vi "Main.vi"() -> ()   [LabVIEW 2018]
doc: "This project is based on the Queued Message Handler template.\n\nThe Event Handling Loop generates messages based on user interface actions.\n\nThe Message Handling Loop processes messages generated by the Event Handling Loop, or by other messages. There are also Acquisition and Logging message handling loop subVIs, and a chart updating loop."
uses:
  Settings/Settings.ctl
  Acquisition/Hardware Configuration.ctl
  Logging/Logging Configuration.ctl
  controls/UI RefNums.ctl
  Analysis/Global Tube Length.vi
  support/Global Offsets.vi
  Settings/Settings.lvlib
  support/User Event - Stop/User Event - Stop.lvlib
  support/Message Queue/Message Queue.lvlib
  <vilib>/Analysis/NI_AALBase.lvlib
  Logging/Logging.lvlib
  Analysis/Analysis.lvlib
  Acquisition/Acquisition.lvlib
panel:
  out "Long Offset":string
  out "Mid Offset":string
  out "Short Offset":string
  out "Timer":dbl(knob) scale=0.0..300.0
  in  "Long":dbl format="%_5g"
  in  "Mid":dbl format="%_5g"
  in  "Short":dbl format="%.4g"
  out "System Log":string
  out "L":bool
  out "M":bool
  in  "Collar":dbl format="%.4g"
  out "Thermistors":cluster{i32[], "Temp Out":dbl[]}(graph)
  in  "Exit":bool
  in  "Settings":bool
  out "RS232 Buffer":string
  out "S":bool
  in  "Start":bool
  out "Average Temperature Time Series":dbl(graph)
  out "Ring Time":waveform(dbl)(graph)
  # "Offsets"
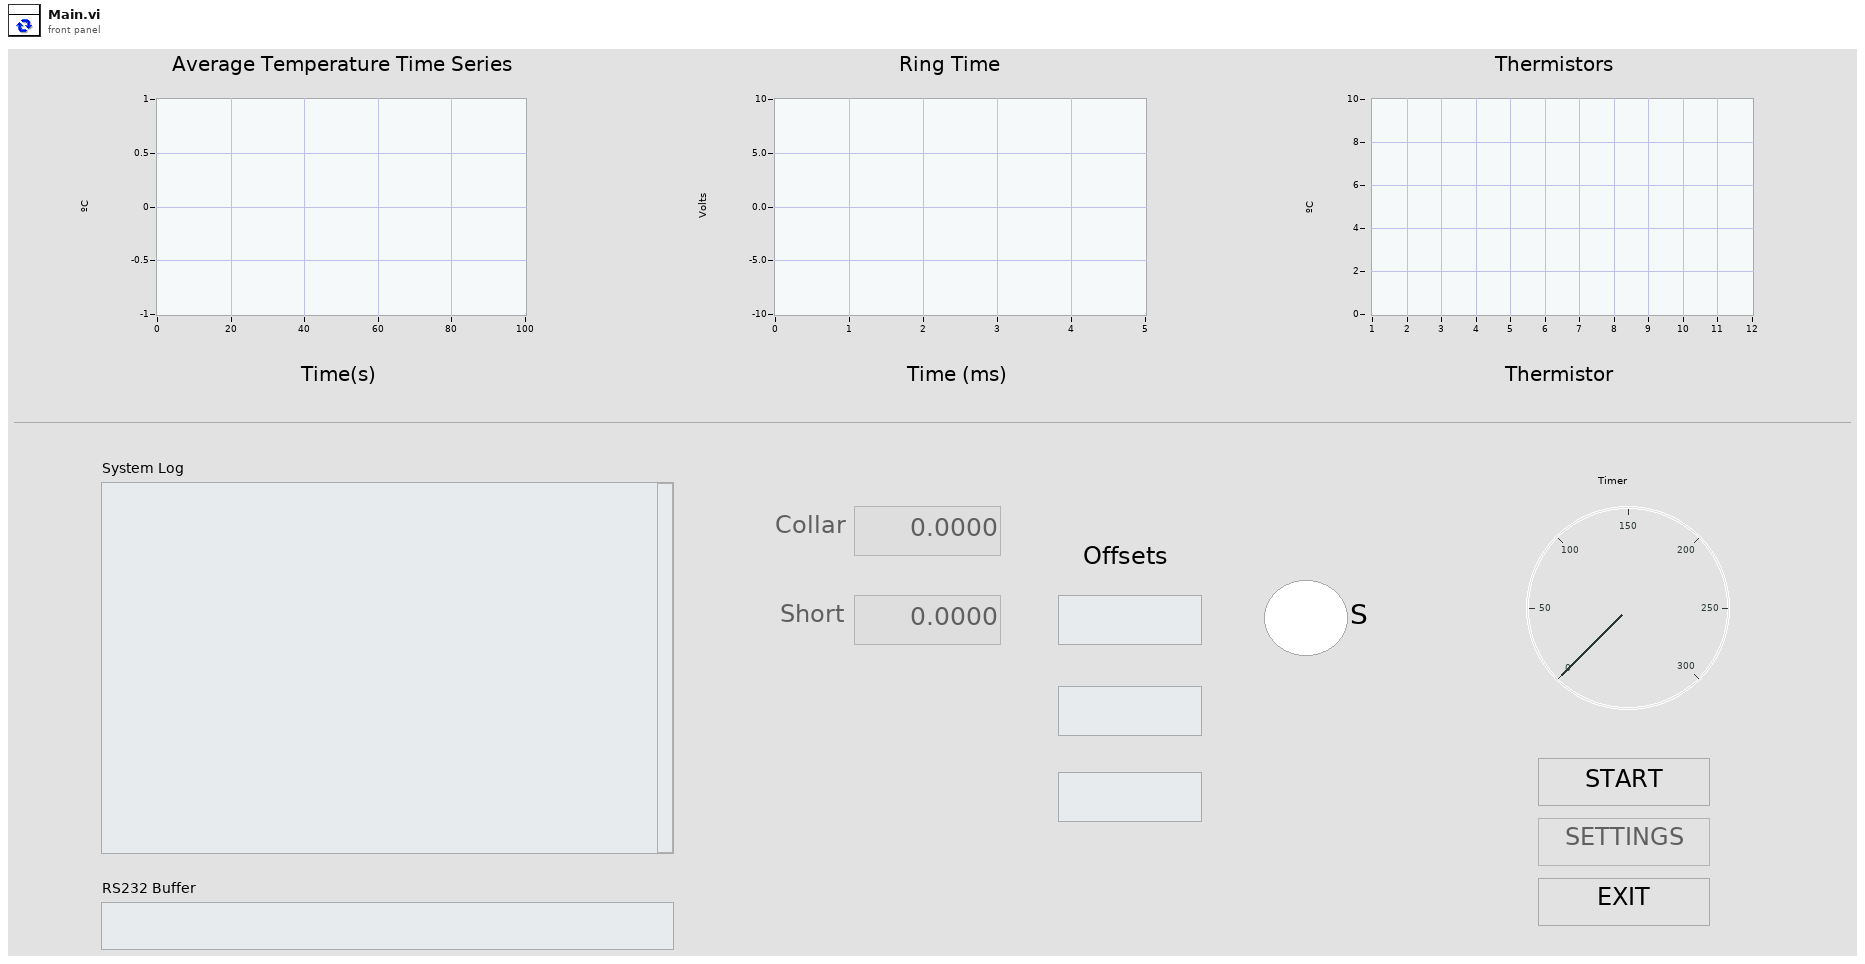
[diagram p1: front panel]
types:
  T1 = typedef "Settings.ctl" = cluster{"Hardware Configuration":T2, "Logging Configuration":T3, "UI RefNums":T4, "Meta Data":cluster{"Calibration Location":string, "Operator Name":string, "Sensor SN":string, "Cal Tube SN":string, "Comments":string, "Start Time":string}}
  T2 = typedef "Acquisition.lvlib/Hardware Configuration.ctl" = cluster{"DAQmx AI Channels":tag, "Aquatrak COM Port":refnum<visa-resource-name>, "Ring Time Task":refnum<k21>}
  T3 = typedef "Logging.lvlib/Logging Configuration.ctl" = cluster{"Log File Base Path":path, "Data Log Refnum":refnum<k1>}
  T4 = typedef "UI RefNums.ctl" = cluster{"Start Ref":refnum<vi>, "Settings Ref":refnum<vi>, "Exit Ref":refnum<vi>, "System Log Ref":refnum<vi>, "RS232 Buffer Ref":refnum<vi>, "Ringtime Ref":refnum<vi>, "Avg Temp Ref":refnum<vi>, "Thermistors Ref":refnum<vi>, "Collar Meas Ref":refnum<vi>, "Short Meas Ref":refnum<vi>, "Mid Meas Ref":refnum<vi>, "Long Meas Ref":refnum<vi>, "Short LED Ref":refnum<vi>, "Mid LED Ref":refnum<vi>, "Long LED Ref":refnum<vi>, "Short Offset Ref":refnum<vi>, "Mid Offset Ref":refnum<vi>, "Long Offset Ref":refnum<vi>, "Timer Ref":refnum<vi>}
  T5 = typedef "Message Queue.lvlib/All Message Queues.ctl" = cluster{"UI":refnum<queue>, "Acquisition":refnum<queue>, "Logging":refnum<queue>, "Analyze":refnum<queue>, "Data Notifier":refnum<notifier>, "Data Queue":refnum<queue>}
  T6 = typedef "Acquired Data.ctl" = cluster{"Average Range":dbl, "Temp Array":dbl[][], "Cal Counts":i32, "Range Counts":i32, "Timestamp (UTC)":string}
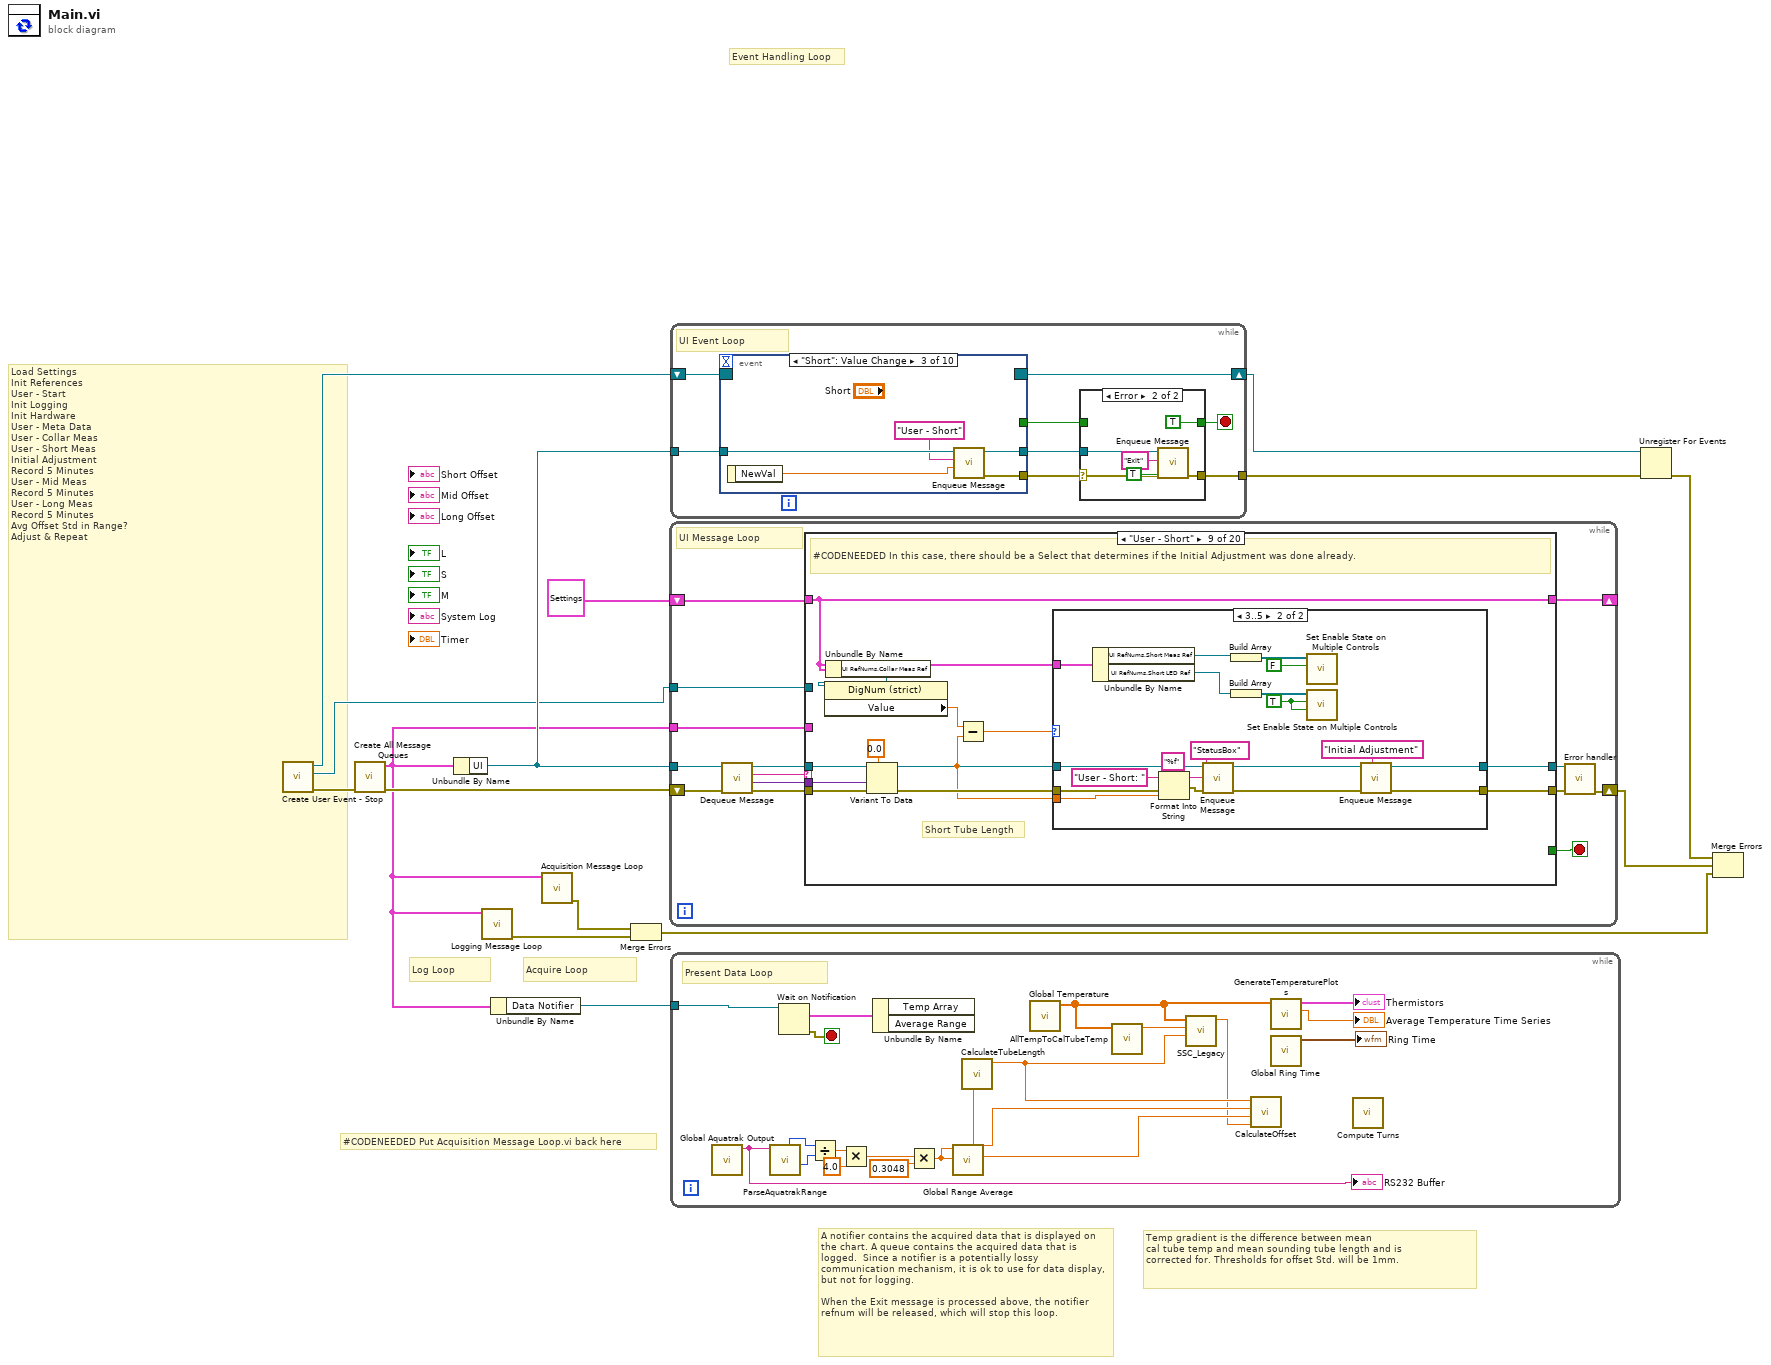
[diagram p0: block diagram]
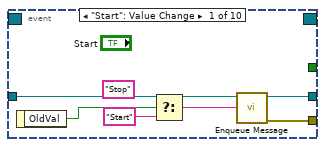
[diagram p3: hidden frame]
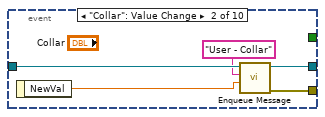
[diagram p4: hidden frame]
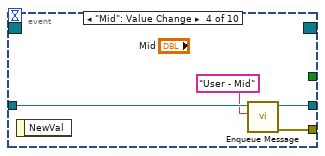
[diagram p5: hidden frame]
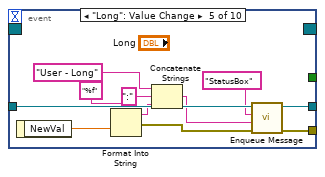
[diagram p6: hidden frame]
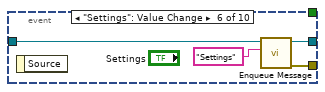
[diagram p7: hidden frame]
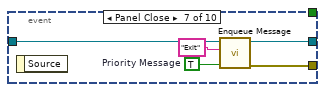
[diagram p8: hidden frame]
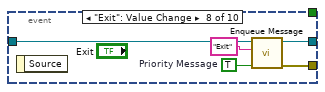
[diagram p9: hidden frame]
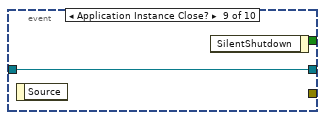
[diagram p10: hidden frame]
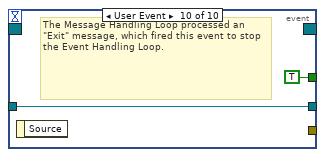
[diagram p11: hidden frame]
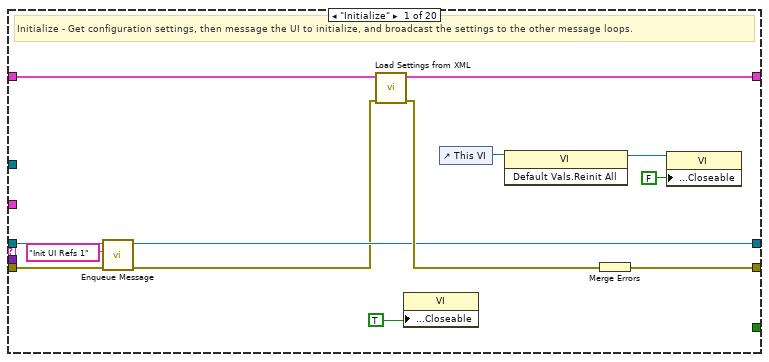
[diagram p12: hidden frame]
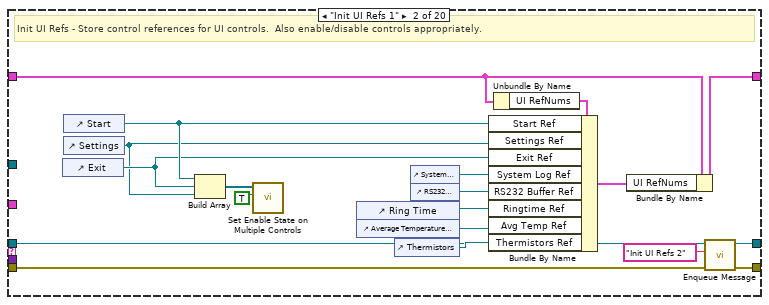
[diagram p13: hidden frame]
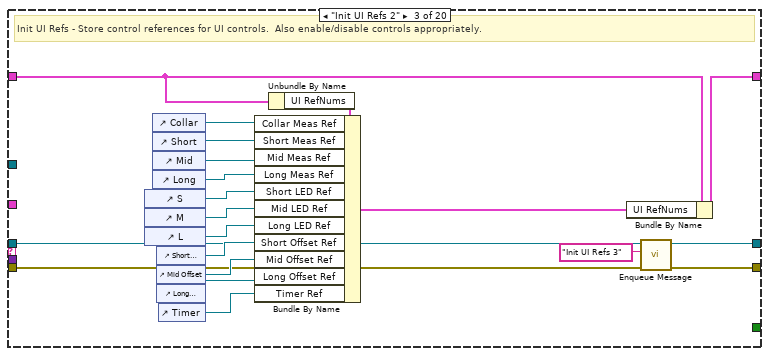
[diagram p14: hidden frame]
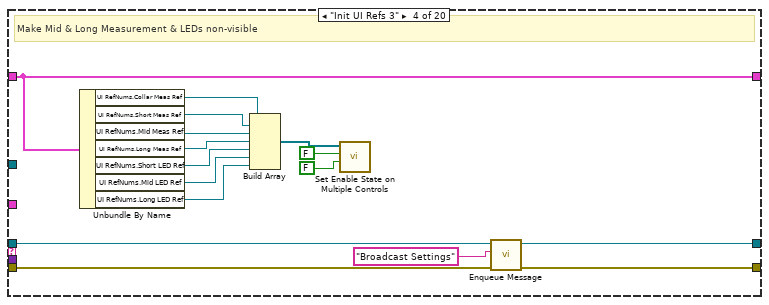
[diagram p15: hidden frame]
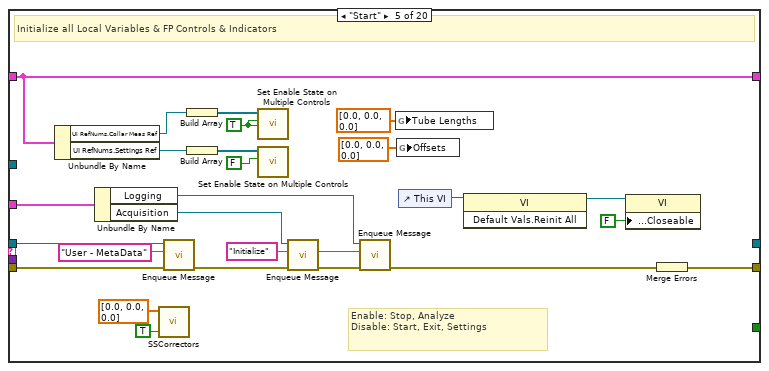
[diagram p16: hidden frame]
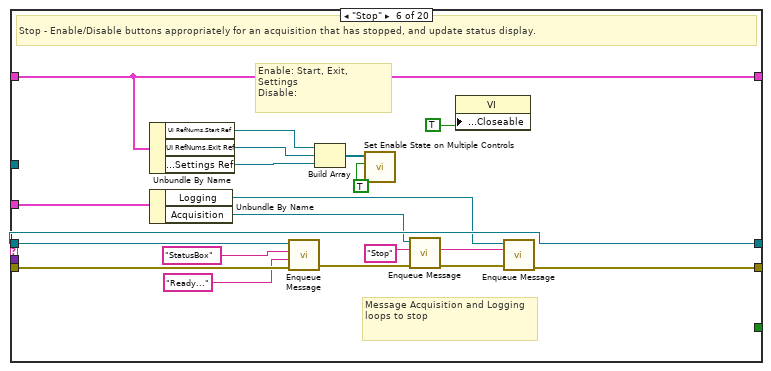
[diagram p17: hidden frame]
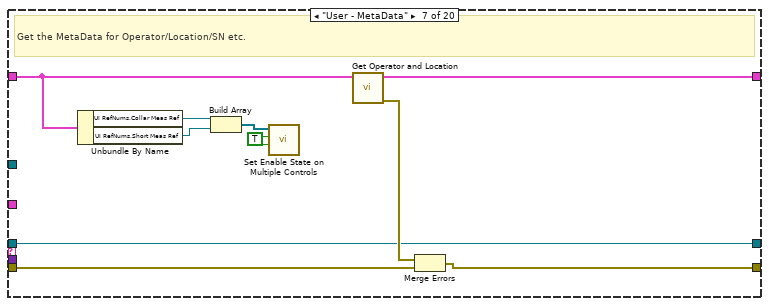
[diagram p18: hidden frame]
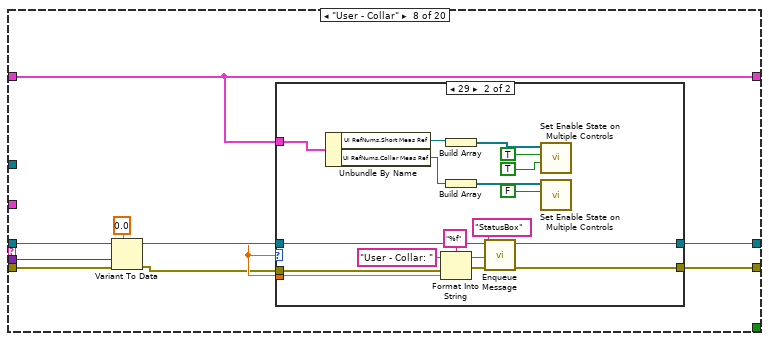
[diagram p19: hidden frame]
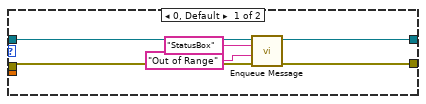
[diagram p20: hidden frame]
diagram:
  # "#CODENEEDED Put Acquisition Message Loop.vi back here"
  # "Acquire Loop"
  # "Log Loop"
  # "Event Handling Loop"
  # "Temp gradient is the difference between mean\ncal tube temp and mean sounding tube length and is \ncorrected for. Thresholds for offset Std. will be 1mm."
  # "A notifier contains the acquired data that is displayed on the chart. A queue contains the acquired data that is logged.  Since a notifier is a potentially lossy communication mechanism, it is ok to use for data display, but not for logging.\n\nWhen the Exit message is processed above, the notifier refnum will be released, which will stop this loop."
  # "Load Settings\nInit References\nUser - Start\nInit Logging\nInit Hardware\nUser - Meta Data\nUser - Collar Meas\nUser - Short Meas\nInitial Adjustment\nRecord 5 Minutes\nUser - Mid Meas\nRecord 5 Minutes\nUser - Long Meas\nRecord 5 Minutes\nAvg Offset Std in Range?\nAdjust & Repeat"
  n1 = call "Create User Event - Stop.vi"() -> ("error out"=w11:errorcluster, "User Event - Stop"=w5:refnum<user-event>, "Stop Event Registration Refnum"=w12:refnum<event-registration>)  [unwired: 9 in]
  n2 = call "Create All Message Queues.vi"("error in (no error)"=w11) -> ("error out"=w8:errorcluster, "Message Queues out"=w2:T5)  [unwired: 9 in]
  n3 = Unbundle By Name(w2) -> ("UI"=w15:refnum<queue>)
  n4 = call "Logging Message Loop.vi"("Message Queues"=w2) -> ("error out"=w4:errorcluster)  [unwired: 10 in]
  n5 = Unbundle By Name(w2) -> ("Data Notifier"=w6:refnum<notifier>)
  n6 = call "Acquisition Message Loop.vi"("Message Queues"=w2) -> ("error out"=w1:errorcluster)  [unwired: 10 in]
  n7 = Merge Errors(w1, w4) -> (w3:errorcluster)
  n8 = while {
    tunnel: w15 -> [w22]
    tunnel: w5 -> [w28]
    shift-right: [w19] -> w14
    shift-left: w8 -> [w27]
    shift-right: [w17] -> _
    shift-left: T1 {"Hardware Configuration"={"DAQmx AI Channels"="", "Aquatrak COM Port"="", "Ring Time Task"=""}, "Logging Configuration"={"Log File Base Path"=path "", "Data Log Refnum"=refnum}, "UI RefNums"={"Start Ref"=refnum, "Settings Ref"=refnum, "Exit Ref"=refnum, "System Log Ref"=refnum, "RS232 Buffer Ref"=refnum, "Ringtime Ref"=refnum, "Avg Temp Ref"=refnum, "Thermistors Ref"=refnum, "Collar Meas Ref"=refnum, "Short Meas Ref"=refnum, "Mid Meas Ref"=refnum, "Long Meas Ref"=refnum, "Short LED Ref"=refnum, "Mid LED Ref"=refnum, "Long LED Ref"=refnum, "Short Offset Ref"=refnum, "Mid Offset Ref"=refnum, "Long Offset Ref"=refnum, "Timer Ref"=refnum}, "Meta Data"={"Calibration Location"="", "Operator Name"="", "Sensor SN"="", "Cal Tube SN"="", "Comments"="", "Start Time"=""}} ("Settings") -> [w21]
    tunnel: w2 -> [w16]
    stop <- w29 stop-if-true
    # "UI Message Loop"
    n9 = call "Dequeue Message.vi"("error in (no error)"=w27, "Message Queue"=w22) -> ("error out"=w26:errorcluster, "Message Data"=w24:variant, "Message"=w25:string, "dup Message Queue"=w23:refnum<queue>)  [unwired: 6 in]
    n10 = case "Message Cases" shown="\"User - Short\"" w25 {
      selector: w25 -> [_ _ _ _ _ _ _ _ _ _ _ _ _ _ _ _ _ _ _ w367]
      tunnel: w23 -> [w39 w46 w65 w91 w109 w140 w146 w159 w195 w228 w238 w265 w304 w306 w313 w327 w338 w354 w358 w362]
      tunnel: w26 -> [w38 w45 w64 w90 w108 w139 w149 w156 w192 w223 w235 w268 w305 w308 w316 w331 w339 w350 w361 _]
      tunnel: [w37 w43 w62 w88 w120 w131 w147 w157 w193 w222 w236 w268 w305 w308 w315 w332 w336 w347 w360 w365] -> w18
      tunnel: [_ _ _ _ _ _ _ _ _ _ _ _ _ _ _ _ _ TRUE _ _] -> w29
      tunnel: w24 -> [_ _ _ _ _ _ _ w154 w190 _ w233 _ _ _ _ w330 _ _ _ _]
      tunnel: w28 -> [_ _ _ _ _ _ _ _ _ _ _ _ _ _ _ _ _ w356 _ _]
      tunnel: w21 -> [w42 w55 w80 w97 w113 w127 w144 w151 w186 w226 w231 w270 w303 w307 w312 w326 w340 w355 w359 w363]
      tunnel: [w34 w44 w63 w89 _ w140 w146 w158 w194 w228 w237 w265 w304 w306 w313 w327 w333 _ w358 w362] -> w20
      tunnel: [w40 w54 w79 w97 w113 w127 w148 w151 w186 w226 w231 w270 w303 w307 w312 w326 w335 w355 w359 w363] -> w17
      tunnel: w16 -> [_ _ _ _ w106 w125 _ _ _ w225 _ _ _ _ w311 _ _ w345 _ _]
      frame "Initialize" {
        # "Initialize - Get configuration settings, then message the UI to initialize, and broadcast the settings to the other message loops."
        n11 = call "Enqueue Message.vi"("error in (no error)"=w38, "Message"="Init UI Refs 1", "Message Queue"=w39) -> ("error out"=w33:errorcluster, "dup Message Queue"=w34:refnum<queue>)  [unwired: 7 in]
        n12 = call "Load Settings from XML.vi"("error in (no error)"=w33, "Settings in"=w42) -> ("error out"=w41:errorcluster, "Settings out"=w40:T1)  [unwired: 8 in]
        n13 = property class="VI"("Front Panel.Closeable"=TRUE ("Front Panel Window:Closeable")) -> ()  [unwired: 2 in, 2 out]
        n14 = control-ref of="This VI"() -> (w31:refnum<vi>)
        n15 = invoke class="VI" method="Default Vals.Reinit All"(reference=w31) -> (reference out=w30:refnum<vi>)  [unwired: 2 in, 2 out]
        n16 = Merge Errors(w41) -> (w37:errorcluster)
        n17 = property class="VI"(reference=w30, "Front Panel.Closeable"=FALSE ("Front Panel Window:Closeable")) -> ()  [unwired: 1 in, 2 out]
      }
      frame "Init UI Refs 1" {
        # "Init UI Refs - Store control references for UI controls.  Also enable/disable controls appropriately."
        n18 = control-ref of="Exit"() -> (w58:refnum<vi>)
        n19 = control-ref of="Start"() -> (w59:refnum<vi>)
        n20 = control-ref of="Settings"() -> (w57:refnum<vi>)
        n21 = Build Array(w59, w58, w57) -> (w60:refnum<vi>[])
        n22 = call "Set Enable State on Multiple Controls.vi"("Enable?"=TRUE, "Controls"=w60) -> ()  [unwired: 10 in]
        n23 = control-ref of="Ring Time"() -> (w50:refnum<vi>)
        n24 = control-ref of="Average Temperature Time Series"() -> (w49:refnum<vi>)
        n25 = control-ref of="Thermistors"() -> (w48:refnum<vi>)
        n26 = control-ref of="System Log"() -> (w52:refnum<vi>)
        n27 = control-ref of="RS232 Buffer"() -> (w51:refnum<vi>)
        n28 = Unbundle By Name(w55) -> ("UI RefNums"=w56:T4)
        n29 = Bundle By Name(cluster=w56, "Start Ref"=w59, "Settings Ref"=w57, "Exit Ref"=w58, "System Log Ref"=w52, "RS232 Buffer Ref"=w51, "Ringtime Ref"=w50, "Avg Temp Ref"=w49, "Thermistors Ref"=w48) -> (w53:T4)
        n30 = Bundle By Name(cluster=w55, "UI RefNums"=w53) -> (w54:T1)
        n31 = call "Enqueue Message.vi"("error in (no error)"=w45, "Message"="Init UI Refs 2", "Message Queue"=w46) -> ("error out"=w43:errorcluster, "dup Message Queue"=w44:refnum<queue>)  [unwired: 7 in]
      }
      frame "Init UI Refs 2" {
        # "Init UI Refs - Store control references for UI controls.  Also enable/disable controls appropriately."
        n32 = control-ref of="S"() -> (w77:refnum<vi>)
        n33 = control-ref of="M"() -> (w76:refnum<vi>)
        n34 = control-ref of="L"() -> (w75:refnum<vi>)
        n35 = control-ref of="Collar"() -> (w73:refnum<vi>)
        n36 = control-ref of="Short"() -> (w72:refnum<vi>)
        n37 = control-ref of="Mid"() -> (w71:refnum<vi>)
        n38 = control-ref of="Long"() -> (w70:refnum<vi>)
        n39 = control-ref of="Short Offset"() -> (w69:refnum<vi>)
        n40 = control-ref of="Mid Offset"() -> (w68:refnum<vi>)
        n41 = control-ref of="Long Offset"() -> (w67:refnum<vi>)
        n42 = control-ref of="Timer"() -> (w74:refnum<vi>)
        n43 = Unbundle By Name(w80) -> ("UI RefNums"=w81:T4)
        n44 = Bundle By Name(cluster=w81, "Collar Meas Ref"=w73, "Short Meas Ref"=w72, "Mid Meas Ref"=w71, "Long Meas Ref"=w70, "Short LED Ref"=w77, "Mid LED Ref"=w76, "Long LED Ref"=w75, "Short Offset Ref"=w69, "Mid Offset Ref"=w68, "Long Offset Ref"=w67, "Timer Ref"=w74) -> (w78:T4)
        n45 = Bundle By Name(cluster=w80, "UI RefNums"=w78) -> (w79:T1)
        n46 = call "Enqueue Message.vi"("error in (no error)"=w64, "Message"="Init UI Refs 3", "Message Queue"=w65) -> ("error out"=w62:errorcluster, "dup Message Queue"=w63:refnum<queue>)  [unwired: 7 in]
      }
      frame "Init UI Refs 3" {
        # "Make Mid & Long Measurement & LEDs non-visible"
        n47 = Unbundle By Name(w97) -> ("UI RefNums.Collar Meas Ref"=w82:refnum<vi>, "UI RefNums.Short Meas Ref"=w87:refnum<vi>, "UI RefNums.Mid Meas Ref"=w96:refnum<vi>, "UI RefNums.Long Meas Ref"=w95:refnum<vi>, "UI RefNums.Short LED Ref"=w94:refnum<vi>, "UI RefNums.Mid LED Ref"=w93:refnum<vi>, "UI RefNums.Long LED Ref"=w86:refnum<vi>)
        n48 = Build Array(w82, w87, w96, w95, w94, w93, w86) -> (w84:refnum<vi>[])
        n49 = call "Set Enable State on Multiple Controls.vi"("Visible?"=FALSE ("Enable?"), "Enable?"=FALSE, "Controls"=w84) -> ()  [unwired: 9 in]
        n50 = call "Enqueue Message.vi"("error in (no error)"=w90, "Message"="Broadcast Settings", "Message Queue"=w91) -> ("error out"=w88:errorcluster, "dup Message Queue"=w89:refnum<queue>)  [unwired: 7 in]
      }
      frame "Start" {
        w101 = TRUE ("Enable?")
        w117 = "Initialize" ("Message")
        # "Enable: Stop, Analyze\nDisable: Start, Exit, Settings"
        # "Initialize all Local Variables & FP Controls & Indicators"
        n51 = Unbundle By Name(w113) -> ("UI RefNums.Collar Meas Ref"=w102:refnum<vi>, "UI RefNums.Settings Ref"=w112:refnum<vi>)
        n52 = Unbundle By Name(w106) -> ("Logging"=w105:refnum<queue>, "Acquisition"=w104:refnum<queue>)
        n53 = call "SSCorrectors.vi"("Write?"=TRUE, "SSC In (meters)"=dbl[] [0.0, 0.0, 0.0]) -> ()  [unwired: 8 in, 2 out]
        n54 = call "Enqueue Message.vi"("error in (no error)"=w108, "Message"="User - MetaData", "Message Queue"=w109) -> ("error out"=w107:errorcluster)  [unwired: 7 in, 1 out]
        n55 = Build Array(w102) -> (w103:refnum<vi>[])
        n56 = Build Array(w112) -> (w111:refnum<vi>[])
        n57 = call "Set Enable State on Multiple Controls.vi"("Visible?"=w101, "Enable?"=w101, "Controls"=w103) -> ()  [unwired: 9 in]
        n58 = call "Set Enable State on Multiple Controls.vi"("Enable?"=FALSE, "Controls"=w111) -> ()  [unwired: 10 in]
        n59 = call "Enqueue Message.vi"("error in (no error)"=w107, "Message"=w117, "Message Queue"=w104) -> ("error out"=w118:errorcluster)  [unwired: 7 in, 1 out]
        n60 = call "Enqueue Message.vi"("error in (no error)"=w118, "Message"=w117, "Message Queue"=w105) -> ("error out"=w121:errorcluster)  [unwired: 7 in, 1 out]
        n61 = global write "Global Tube Length.vi" "Tube Lengths"(dbl[] [0.0, 0.0, 0.0] ("Tube Lengths")) -> ()
        n62 = global write "Global Offsets.vi" "Offsets"(dbl[] [0.0, 0.0, 0.0] ("Offsets")) -> ()
        n63 = control-ref of="This VI"() -> (w99:refnum<vi>)
        n64 = invoke class="VI" method="Default Vals.Reinit All"(reference=w99) -> (reference out=w98:refnum<vi>)  [unwired: 2 in, 2 out]
        n65 = property class="VI"(reference=w98, "Front Panel.Closeable"=FALSE ("Front Panel Window:Closeable")) -> ()  [unwired: 1 in, 2 out]
        n66 = Merge Errors(w121) -> (w120:errorcluster)
      }
      frame "Stop" {
        w128 = "Stop" ("Message")
        # "Message Acquisition and Logging loops to stop"
        # "Stop - Enable/Disable buttons appropriately for an acquisition that has stopped, and update status display."
        # "Enable: Start, Exit, Settings\nDisable:"
        n67 = Unbundle By Name(w127) -> ("UI RefNums.Start Ref"=w135:refnum<vi>, "UI RefNums.Exit Ref"=w134:refnum<vi>, "UI RefNums.Settings Ref"=w133:refnum<vi>)
        n68 = Unbundle By Name(w125) -> ("Logging"=w124:refnum<queue>, "Acquisition"=w123:refnum<queue>)
        n69 = call "Enqueue Message.vi"("error in (no error)"=w139, "Message Data"="Ready..." ("Ready..."), "Message"="StatusBox", "Message Queue"=w140) -> ("error out"=w129:errorcluster)  [unwired: 6 in, 1 out]
        n70 = Build Array(w135, w134, w133) -> (w126:refnum<vi>[])
        n71 = call "Set Enable State on Multiple Controls.vi"("Enable?"=TRUE, "Controls"=w126) -> ()  [unwired: 10 in]
        n72 = call "Enqueue Message.vi"("error in (no error)"=w129, "Message"=w128, "Message Queue"=w123) -> ("error out"=w130:errorcluster)  [unwired: 7 in, 1 out]
        n73 = property class="VI"("Front Panel.Closeable"=TRUE ("Front Panel Window:Closeable")) -> ()  [unwired: 2 in, 2 out]
        n74 = call "Enqueue Message.vi"("error in (no error)"=w130, "Message"=w128, "Message Queue"=w124) -> ("error out"=w131:errorcluster)  [unwired: 7 in, 1 out]
      }
      frame "User - MetaData" {
        w141 = TRUE ("Enable?")
        # "Get the MetaData for Operator/Location/SN etc."
        n75 = Unbundle By Name(w144) -> ("UI RefNums.Collar Meas Ref"=w143:refnum<vi>, "UI RefNums.Short Meas Ref"=w142:refnum<vi>)
        n76 = Build Array(w143, w142) -> (w145:refnum<vi>[])
        n77 = call "Set Enable State on Multiple Controls.vi"("Visible?"=w141, "Enable?"=w141, "Controls"=w145) -> ()  [unwired: 9 in]
        n78 = call "Get Operator and Location.vi"("Settings in"=w144) -> ("error out"=w150:errorcluster, "Settings"=w148:T1)  [unwired: 9 in]
        n79 = Merge Errors(w150, w149) -> (w147:errorcluster)
      }
      frame "User - Collar" {
        n80 = Variant To Data(error in=w156, type=0.0, Variant=w154) -> (data=w153:dbl, error out=w152:errorcluster)
        n81 = case shown="29" w153 {
          tunnel: w159 -> [w164 w182]
          tunnel: [w163 w178] -> w158
          tunnel: [w162 w177] -> w157
          tunnel: w153 -> [_ w180]
          tunnel: w152 -> [w161 w174]
          tunnel: w151 -> [_ w173]
          frame 0, Default {
            n82 = call "Enqueue Message.vi"("error in (no error)"=w161, "Message Data"="Out of Range" ("Message"), "Message"="StatusBox", "Message Queue"=w164) -> ("error out"=w162:errorcluster, "dup Message Queue"=w163:refnum<queue>)  [unwired: 6 in]
          }
          frame 29 {
            n83 = Unbundle By Name(w173) -> ("UI RefNums.Short Meas Ref"=w169:refnum<vi>, "UI RefNums.Collar Meas Ref"=w166:refnum<vi>)
            n84 = Format Into String(format string="%f" ("Message"), initial string="User - Collar: " ("Message"), error in=w174, w180) -> (resulting string=w176:string, error out=w175:errorcluster)
            n85 = Build Array(w169) -> (w171:refnum<vi>[])
            n86 = Build Array(w166) -> (w168:refnum<vi>[])
            n87 = call "Enqueue Message.vi"("error in (no error)"=w175, "Message Data"=w176, "Message"="StatusBox", "Message Queue"=w182) -> ("error out"=w177:errorcluster, "dup Message Queue"=w178:refnum<queue>)  [unwired: 6 in]
            n88 = call "Set Enable State on Multiple Controls.vi"("Visible?"=TRUE ("Enable?"), "Enable?"=TRUE, "Controls"=w171) -> ()  [unwired: 9 in]
            n89 = call "Set Enable State on Multiple Controls.vi"("Enable?"=FALSE, "Controls"=w168) -> ()  [unwired: 10 in]
          }
        }
      }
      frame "User - Short" {
        # "Short Tube Length"
        # "#CODENEEDED In this case, there should be a Select that determines if the Initial Adjustment was done already."
        n90 = Unbundle By Name(w186) -> ("UI RefNums.Collar Meas Ref"=w185:refnum<vi>)
        n91 = property class="DigNum (strict)"(reference=w185) -> ("Value"=w184:dbl)  [unwired: 1 in, 2 out]
        n92 = Variant To Data(error in=w192, type=0.0, Variant=w190) -> (data=w188:dbl, error out=w189:errorcluster)
        n93 = Subtract(x=w184, y=w188) -> (x-y=w187:dbl)
        n94 = case shown="3..5" w187 {
          tunnel: w195 -> [w200 w220]
          tunnel: [w199 w202] -> w194
          tunnel: [w198 w203] -> w193
          tunnel: w188 -> [_ w218]
          tunnel: w189 -> [w197 w214]
          tunnel: w186 -> [_ w213]
          frame 0, Default {
            n95 = call "Enqueue Message.vi"("error in (no error)"=w197, "Message Data"="Out of Range" ("Message"), "Message"="StatusBox", "Message Queue"=w200) -> ("error out"=w198:errorcluster, "dup Message Queue"=w199:refnum<queue>)  [unwired: 6 in]
          }
          frame 3..5 {
            w204 = TRUE ("Enable?")
            n96 = Unbundle By Name(w213) -> ("UI RefNums.Short Meas Ref"=w210:refnum<vi>, "UI RefNums.Short LED Ref"=w205:refnum<vi>)
            n97 = Format Into String(format string="%f" ("Message"), initial string="User - Short: " ("Message"), error in=w214, w218) -> (resulting string=w216:string, error out=w215:errorcluster)
            n98 = call "Enqueue Message.vi"("error in (no error)"=w215, "Message Data"=w216, "Message"="StatusBox", "Message Queue"=w220) -> ("error out"=w207:errorcluster, "dup Message Queue"=w209:refnum<queue>)  [unwired: 6 in]
            n99 = Build Array(w210) -> (w211:refnum<vi>[])
            n100 = Build Array(w205) -> (w206:refnum<vi>[])
            n101 = call "Set Enable State on Multiple Controls.vi"("Enable?"=FALSE, "Controls"=w211) -> ()  [unwired: 10 in]
            n102 = call "Set Enable State on Multiple Controls.vi"("Visible?"=w204, "Enable?"=w204, "Controls"=w206) -> ()  [unwired: 9 in]
            n103 = call "Enqueue Message.vi"("error in (no error)"=w207, "Message"="Initial Adjustment", "Message Queue"=w209) -> ("error out"=w203:errorcluster, "dup Message Queue"=w202:refnum<queue>)  [unwired: 7 in]
          }
        }
      }
      frame "Initial Adjustment" {
        # "Use Cal Cts & Temperature to Adjust To 4ft"
        # "Alert the Acquisition & Logging Loop"
        # "When Short tube is attached, the initial adjustment uses Avg Temperature and Cal Cts\nto adjust an Aquatrak sensor to approximately the correct location."
        n104 = Unbundle By Name(w225) -> ("Acquisition"=w224:refnum<queue>)
        n105 = call "Enqueue Message.vi"("error in (no error)"=w223, "Message"="Initial Adjustment", "Message Queue"=w224) -> ("error out"=w222:errorcluster)  [unwired: 7 in, 1 out]
      }
      frame "User - Mid" {
        # "Short Tube Length"
        n106 = Variant To Data(error in=w235, type=0.0, Variant=w233) -> (data=w230:dbl, error out=w232:errorcluster)
        n107 = Subtract(x=w230, y=w230) -> (x-y=w229:dbl)
        n108 = case shown="29" w229 {
          tunnel: w238 -> [w243 w263]
          tunnel: [w242 w251] -> w237
          tunnel: [w241 w248] -> w236
          tunnel: w230 -> [_ w261]
          tunnel: w232 -> [w240 w257]
          tunnel: w231 -> [_ w256]
          frame 0, Default {
            n109 = call "Enqueue Message.vi"("error in (no error)"=w240, "Message Data"="Out of Range" ("Message"), "Message"="StatusBox", "Message Queue"=w243) -> ("error out"=w241:errorcluster, "dup Message Queue"=w242:refnum<queue>)  [unwired: 6 in]
          }
          frame 29 {
            w245 = TRUE ("Enable?")
            n110 = Unbundle By Name(w256) -> ("UI RefNums.Mid Meas Ref"=w253:refnum<vi>, "UI RefNums.Mid LED Ref"=w246:refnum<vi>)
            n111 = Format Into String(format string="%f" ("Message"), initial string="User - Mid: " ("Message"), error in=w257, w261) -> (resulting string=w259:string, error out=w258:errorcluster)
            n112 = call "Enqueue Message.vi"("error in (no error)"=w258, "Message Data"=w259, "Message"="StatusBox", "Message Queue"=w263) -> ("error out"=w249:errorcluster, "dup Message Queue"=w252:refnum<queue>)  [unwired: 6 in]
            n113 = Build Array(w253) -> (w254:refnum<vi>[])
            n114 = Build Array(w246) -> (w247:refnum<vi>[])
            n115 = call "Set Enable State on Multiple Controls.vi"("Enable?"=FALSE, "Controls"=w254) -> ()  [unwired: 10 in]
            n116 = call "Set Enable State on Multiple Controls.vi"("Visible?"=w245, "Enable?"=w245, "Controls"=w247) -> ()  [unwired: 9 in]
            n117 = call "Enqueue Message.vi"("error in (no error)"=w249, "Message"="Offset", "Message Queue"=w252) -> ("error out"=w248:errorcluster, "dup Message Queue"=w251:refnum<queue>)  [unwired: 7 in]
          }
        }
      }
      frame "Offset" {
        # "#CODENEEDED Case Structure below has different cases based on Tube Length"
        n118 = case shown="5..7" 0 {
          selector: 0 -> [w272 _ w283 w293]
          tunnel: [_ errorcluster {"status"=FALSE, "code"=0, "source"=""} ("error out") _ _] -> w267
          frame 8..10 {
            n119 = call "SSCorrectors.vi"() -> ("Error Out"=w276:errorcluster, "SSC Out (meters)"=w277:dbl[])  [unwired: 10 in]
            n120 = Replace Array Subset(array=w277, new element=w272, index=2) -> (w279:dbl[])
            n121 = Multiply(x=10000.0, y=w272) -> (x*y=w273:dbl)
            n122 = call "SSCorrectors.vi"("Error In"=w276, "Write?"=TRUE, "SSC In (meters)"=w279) -> ()  [unwired: 7 in, 2 out]
            n123 = case shown="-1250..-970" w273 {
              tunnel: [FALSE TRUE] -> _
              frame 0, Default {
              }
              frame -1250..-970 {
              }
            }
          }
          frame 0, Default {
          }
          frame 2..4 {
            n124 = call "SSCorrectors.vi"() -> ("Error Out"=w289:errorcluster, "SSC Out (meters)"=w288:dbl[])  [unwired: 10 in]
            n125 = Replace Array Subset(array=w288, new element=w283, index=0) -> (w286:dbl[])
            n126 = call "SSCorrectors.vi"("Error In"=w289, "Write?"=TRUE, "SSC In (meters)"=w286) -> ()  [unwired: 7 in, 2 out]
            n127 = Multiply(x=10000.0, y=w283) -> (x*y=w284:dbl)
            n128 = case shown="-1250..-970" w284 {
              tunnel: [FALSE TRUE] -> _
              frame 0, Default {
              }
              frame -1250..-970 {
              }
            }
          }
          frame 5..7 {
            n129 = call "SSCorrectors.vi"() -> ("Error Out"=w299:errorcluster, "SSC Out (meters)"=w298:dbl[])  [unwired: 10 in]
            n130 = Replace Array Subset(array=w298, new element=w293, index=1) -> (w296:dbl[])
            n131 = call "SSCorrectors.vi"("Error In"=w299, "Write?"=TRUE, "SSC In (meters)"=w296) -> ()  [unwired: 7 in, 2 out]
            n132 = Multiply(x=10000.0, y=w293) -> (x*y=w295:dbl)
            n133 = case shown="0, Default" w295 {
              tunnel: [FALSE TRUE] -> _
              frame 0, Default {
              }
              frame -1250..-970 {
              }
            }
          }
        }
        n134 = case shown="No Error" w267 {
          tunnel: [_ dbl[] [0.0, 0.0, 0.0]] -> w269
          frame No Error {
          }
          frame Error {
          }
        }
        n135 = call <vilib>:"Std Deviation and Variance.vi"("X"=w269) -> ()  [unwired: 1 in, 3 out]
      }
      frame "Save" {
        n136 = call "BuildSavePath.vi"("Settings"=w303) -> ()  [unwired: 8 in, 3 out]
        n137 = call "Global Temperature.vi"() -> ()  [unwired: 10 in, 2 out]
        n138 = call "SSCorrectors.vi"() -> ()  [unwired: 10 in, 2 out]
        n139 = call "GenerateAquatrakCalibrationSheet.vi"() -> ()  [unwired: 11 in, 1 out]
      }
      frame "Launch Analysis" {
        n140 = call "AnalyzeCalibrations.vi"() -> ()  [unwired: 12 in]
      }
      frame "Broadcast settings" {
        w314 = "Update Settings" ("Message")
        # "Send the 'Update Settings' message to the Logging and Acqusition message loops."
        n141 = Unbundle By Name(w311) -> ("Logging"=w310:refnum<queue>, "Acquisition"=w309:refnum<queue>)
        n142 = call "Enqueue Message.vi"("error in (no error)"=w316, "Message Data"=w312, "Message"=w314, "Message Queue"=w309) -> ("error out"=w317:errorcluster)  [unwired: 6 in, 1 out]
        n143 = call "Enqueue Message.vi"("error in (no error)"=w317, "Message Data"=w312, "Message"=w314, "Message Queue"=w310) -> ("error out"=w315:errorcluster)  [unwired: 6 in, 1 out]
      }
      frame "StatusBox" {
        # "Update Display - Convert the message data to a string to display in the Status indicator."
        n144 = Unbundle By Name(w326) -> ("UI RefNums.System Log Ref"=w324:refnum<vi>)
        n145 = Variant To Data(error in=w331, type="", Variant=w330) -> (data=w322:string, error out=w328:errorcluster)
        n146 = property class="Str"(reference=w324) -> (reference out=w320:refnum<vi>, "Value"=w323:string)  [unwired: 1 in, 1 out]
        n147 = Concatenate Strings(w323, "\n", w322) -> (w319:string)
        n148 = property class="Str"(reference=w320, "Value"=w319) -> (reference out=w318:refnum<vi>)  [unwired: 1 in, 1 out]
        n149 = String Length(string=w319) -> (length=w325:i32)
        n150 = property class="Str"(reference=w318, "Text.Scroll Position"=w325) -> ()  [unwired: 1 in, 2 out]
        n151 = Merge Errors(w328) -> (w332:errorcluster)
      }
      frame "Settings" {
        # "Launch the Settings Dialog when the user clicks the 'Settings' button."
        n152 = call "Settings Dialog.vi"("error in (no error)"=w339, "Settings in"=w340) -> ("error out"=w337:errorcluster, "Settings out"=w335:T1)  [unwired: 6 in, 2 out]
        n153 = call "Enqueue Message.vi"("error in (no error)"=w337, "Message"="Broadcast Settings", "Message Queue"=w338) -> ("error out"=w336:errorcluster, "dup Message Queue"=w333:refnum<queue>)  [unwired: 7 in]
      }
      frame "Exit" {
        w346 = "Exit" ("Message")
        # "Don't check the error outs. The acquisition and logging queues may have already been released."
        # "Close references owned by the Main VI."
        # "Stop the VI"
        # "Exit - Fire the User Event to stop the Event Handling Loop.  Also send Exit messages to the Acqusition, Analyze and Logging loops."
        n154 = call "Fire User Event - Stop.vi"("User Event - Stop"=w356) -> ("error out"=w349:errorcluster)  [unwired: 10 in]
        n155 = Unbundle By Name(w345) -> ("Logging"=w344:refnum<queue>, "Acquisition"=w343:refnum<queue>, "Data Queue"=w341:refnum<queue>, "Data Notifier"=w342:refnum<notifier>)
        n156 = Merge Errors(w349, w350) -> (w351:errorcluster)
        n157 = Release Queue(queue=w354, error in (no error)=w351) -> (error out=w353:errorcluster)  [unwired: 1 in, 2 out]
        n158 = Release Notifier(notifier=w342, error in (no error)=w353) -> (error out=w352:errorcluster)  [unwired: 1 in, 2 out]
        n159 = Release Queue(queue=w341, error in (no error)=w352) -> (error out=w348:errorcluster)  [unwired: 1 in, 2 out]
        n160 = call "Enqueue Message.vi"("Message"=w346, "Message Queue"=w344) -> ()  [unwired: 8 in, 2 out]
        n161 = call "Enqueue Message.vi"("Message"=w346, "Message Queue"=w343) -> ()  [unwired: 8 in, 2 out]
        n162 = Merge Errors(w348) -> (w347:errorcluster)
      }
      frame "---Copy This Frame---" {
        # "Duplicate this frame when creating new messages.  Change this comment in the duplicated frame to describe this message."
        n163 = Merge Errors(w361) -> (w360:errorcluster)
      }
      frame Default {
        # "'Default' case only runs if there is a message that isn't defined in any of the other cases.  Output a programming error."
        n164 = Format Into String(format string="The invalid message string \"%s\" was received in the Message Handling Loop." ("Invalid Message Loop Message"), w367) -> (resulting string=w364:string)  [unwired: 2 in, 1 out]
        n165 = call <vilib>:"Error Cluster From Error Code.vi"("error message (\"\")"=w364, "error code (0)"=1) -> ("error out"=w365:errorcluster)  [unwired: 7 in]
      }
    }
    n166 = call "Error handler.vi"("error in (no error)"=w18, "Queue in"=w20) -> ("error out"=w19:errorcluster)  [unwired: 9 in]
  }
  n167 = while {
    tunnel: w15 -> [w372]
    tunnel: [w370] -> w13
    shift-right: [w371] -> w9
    shift-left: w12 -> [w373]
    stop <- w375 stop-if-true
    # "UI Event Loop"
    n168 = event shown="[2] \"Short\": Value Change" {
      selector: w373 -> [_ _ _ _ _ _ _ _ _ _]
      dyn-events: [_ _ _ _ _ _ _ _ _ _] -> w371
      timeout: _ -> [_ _ _ _ _ _ _ _ _ _]
      tunnel: [_ _ _ _ _ _ _ _ _ TRUE ("Discard?")] -> w376
      tunnel: w372 -> [w390 w395 w400 w404 w415 w418 w422 w427 w431 w432]
      tunnel: [w391 w396 w401 w405 w416 w420 w425 w430 _ _] -> w374
      tunnel: [w385 w392 w398 w402 w406 w417 w421 w426 w431 w432] -> w369
      event "Start": Value Change {
        n169 = event-data() -> ("OldVal"=w389:bool)  [unwired: 1 in]
        n170 = Select(t="Stop" ("Message"), s=w389, f="Start" ("Message")) -> (s? t:f=w386:string)
        n171 = call "Enqueue Message.vi"("Message"=w386, "Message Queue"=w390) -> ("error out"=w391:errorcluster, "dup Message Queue"=w385:refnum<queue>)  [unwired: 8 in]
      }
      event "Collar": Value Change {
        n172 = event-data() -> ("NewVal"=w393:dbl)  [unwired: 1 in]
        n173 = call "Enqueue Message.vi"("Message Data"=w393, "Message"="User - Collar", "Message Queue"=w395) -> ("error out"=w396:errorcluster, "dup Message Queue"=w392:refnum<queue>)  [unwired: 7 in]
      }
      event "Short": Value Change {
        n174 = event-data() -> ("NewVal"=w397:dbl)  [unwired: 1 in]
        n175 = call "Enqueue Message.vi"("Message Data"=w397, "Message"="User - Short", "Message Queue"=w400) -> ("error out"=w401:errorcluster, "dup Message Queue"=w398:refnum<queue>)  [unwired: 7 in]
      }
      event "Mid": Value Change {
        n176 = event-data() -> ()  [unwired: 1 in, 1 out]
        n177 = call "Enqueue Message.vi"("Message"="User - Mid", "Message Queue"=w404) -> ("error out"=w405:errorcluster, "dup Message Queue"=w402:refnum<queue>)  [unwired: 8 in]
      }
      event "Long": Value Change {
        n178 = event-data() -> ("NewVal"=w412:dbl)  [unwired: 1 in]
        n179 = Format Into String(format string="%f", w412) -> (resulting string=w409:string, error out=w414:errorcluster)  [unwired: 2 in]
        n180 = Concatenate Strings("User - Long" ("Message"), ":", w409) -> (w410:string)
        n181 = call "Enqueue Message.vi"("error in (no error)"=w414, "Message Data"=w410, "Message"="StatusBox", "Message Queue"=w415) -> ("error out"=w416:errorcluster, "dup Message Queue"=w406:refnum<queue>)  [unwired: 6 in]
      }
      event "Settings": Value Change {
        n182 = event-data() -> ()  [unwired: 1 in, 1 out]
        n183 = call "Enqueue Message.vi"("Message"="Settings", "Message Queue"=w418) -> ("error out"=w420:errorcluster, "dup Message Queue"=w417:refnum<queue>)  [unwired: 8 in]
      }
      event Panel Close {
        w423 = TRUE  # Priority Message
        n184 = event-data() -> ()  [unwired: 1 in, 1 out]
        n185 = call "Enqueue Message.vi"("Priority Message? (F)"=w423, "Message"="Exit", "Message Queue"=w422) -> ("error out"=w425:errorcluster, "dup Message Queue"=w421:refnum<queue>)  [unwired: 7 in]
      }
      event "Exit": Value Change {
        w428 = TRUE  # Priority Message
        n186 = event-data() -> ()  [unwired: 1 in, 1 out]
        n187 = call "Enqueue Message.vi"("Priority Message? (F)"=w428, "Message"="Exit", "Message Queue"=w427) -> ("error out"=w430:errorcluster, "dup Message Queue"=w426:refnum<queue>)  [unwired: 7 in]
      }
      event Application Instance Close? {
        n188 = event-data() -> ()  [unwired: 1 in, 1 out]
        n189 = event-data() -> ()  [unwired: 2 in, 1 out]
      }
      event User Event {
        # "The Message Handling Loop processed an \"Exit\" message, which fired this event to stop the Event Handling Loop."
        n190 = event-data() -> ()  [unwired: 1 in, 1 out]
      }
    }
    n191 = case shown="Error" w374 {
      selector: w374 -> [w377 w380]
      tunnel: [w378 TRUE ("Discard?")] -> w375
      tunnel: w376 -> [w378 _]
      tunnel: w369 -> [_ w381]
      tunnel: [w377 w379] -> w370
      frame No Error {
      }
      frame Error {
        n192 = call "Enqueue Message.vi"("Priority Message? (F)"=TRUE ("Discard?"), "error in (no error)"=w380, "Message"="Exit", "Message Queue"=w381) -> ("error out"=w379:errorcluster)  [unwired: 6 in, 1 out]
      }
    }
  }
  n193 = while "Data Display Loop" {
    tunnel: w6 -> [w453]
    stop <- w452 stop-if-true
    # "Present Data Loop"
    n194 = call "Global Aquatrak Output.vi"() -> ("AT Out"=w434:string)  [unwired: 9 in, 1 out]
    "RS232 Buffer" <- w434
    n195 = call "ParseAquatrakRange.vi"("Incoming String"=w434) -> ("Cal Counts"=w443:i32, "Range Counts"=w444:i32)  [unwired: 6 in, 3 out]
    n196 = Wait on Notification(notifier=w453) -> (notification=w449:T6, error out=w452:errorcluster)  [unwired: 3 in, 2 out]
    n197 = Divide(x=w444, y=w443) -> (x/y=w442:dbl)
    n198 = Multiply(x=w442, y=4.0) -> (x*y=w439:dbl)
    n199 = Unbundle By Name(w449) -> ()  [unwired: 2 out]
    n200 = Multiply(x=w439, y=0.3048) -> (x*y=w438:dbl)
    n201 = call "Global Range Average.vi"("Range In"=w438) -> ("Std"=w446:dbl, "Average Range"=w447:dbl)  [unwired: 9 in]
    n202 = call "CalculateTubeLength.vi"("Range"=w438) -> ("Tube Length"=w448:dbl)  [unwired: 10 in]
    n203 = call "Global Temperature.vi"() -> ("Temp Out"=w450:dbl[])  [unwired: 10 in, 1 out]
    n204 = call "AllTempToCalTubeTemp.vi"("All Temps"=w450) -> ("Cal Tube Temps"=w451:dbl)  [unwired: 10 in]
    n205 = call "SSC_Legacy.vi"("Tube Length"=w448, "Cal Tube Temp"=w451, "Temp Out"=w450) -> ("SSC Out(m)"=w445:dbl)  [unwired: 8 in]
    n206 = call "CalculateOffset.vi"("SSC"=w445, "Range Std."=w446, "Range"=w447, "Tube Length"=w448) -> ()  [unwired: 6 in, 2 out]
    n207 = call "GenerateTemperaturePlots.vi"("Temp Out"=w450) -> ("mean"=→"Average Temperature Time Series":dbl, "Cluster"=→"Thermistors":cluster{i32[], "Temp Out":dbl[]})  [unwired: 9 in]
    n208 = call "Global Ring Time.vi"() -> ("Ring Time Plot Out"=→"Ring Time":waveform(dbl))  [unwired: 9 in, 1 out]
    n209 = call "Compute Turns.vi"() -> ()  [unwired: 11 in, 1 out]
  }
  n210 = Unregister For Events(event registration refnum=w9, error in=w13) -> (error out=w10:errorcluster)
  n211 = Merge Errors(w10, w14, w3) -> ()  [unwired: 1 out]
